vi "test1.vi"() -> ()   [LabVIEW 2014]
uses:
  <userlib>/ROS for LabVIEW Software/ROS/Code/Console/Servers/ServerSubs/TopicDef.ctl
  <userlib>/ROS for LabVIEW Software/ROS/Code/SubVIs/_ROSDirection.ctl
  <userlib>/ROS for LabVIEW Software/ROS/MessageBuilding/std_msgs/subs/float32Scalar.vi
  <userlib>/ROS for LabVIEW Software/ROS/MessageBuilding/std_msgs/subs/stringScalar.vi
  <userlib>/ROS for LabVIEW Software/ROS/MessageBuilding/std_msgs/subs/u8Scalar.vi
panel:
  in  "Stamp":cluster{"frame_id":string, "reset seq?":bool}={"frame_id"="base_range", "reset seq?"=FALSE}
  in  "Range Data":T1={"Radiation Type"=enum."ultrasound", "Field of View"=2.0, "Min Range (m)"=0.0, "Max Range (m)"=2.0, "Range (m)"=0.0}
  in  "Numeric":sgl
  in  "I said: 2":string="Hello world!"
  out "error out 2":errorcluster
  in  "stop 2":bool
  in  "I said:":string="Hello world!"
  out "error out":errorcluster
  in  "stop":bool
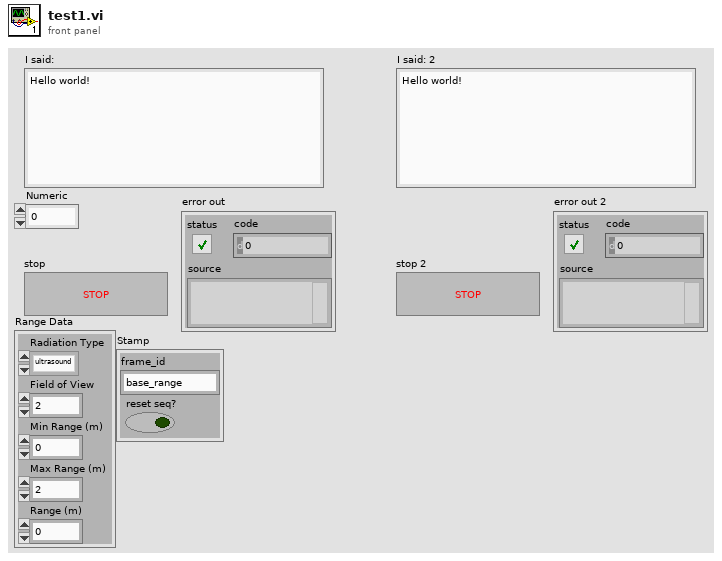
[diagram p1: front panel]
types:
  T1 = cluster{"Radiation Type":enum16{"ultrasound", "infrared"}, "Field of View":sgl, "Min Range (m)":sgl, "Max Range (m)":sgl, "Range (m)":sgl}
  T2 = typedef "TopicDef.ctl" = cluster{"Topic":string, "Type":string, "Action":T3, "Update (ms)":u16, "queue size":u16}
  T3 = typedef "_ROSDirection.ctl" = enum16{"Node", "Publisher", "Subscriber", "ServiceClient", "ServiceProvider"}
  T4 = typedef "_ROSControl.ctl" = cluster{"topic port":u16, "Node":string, "topic":string, "type":string, "node port":u16, "error ":errorcluster, "Direction":T3, "Update (ms)":u16, "FIFO size":u16}
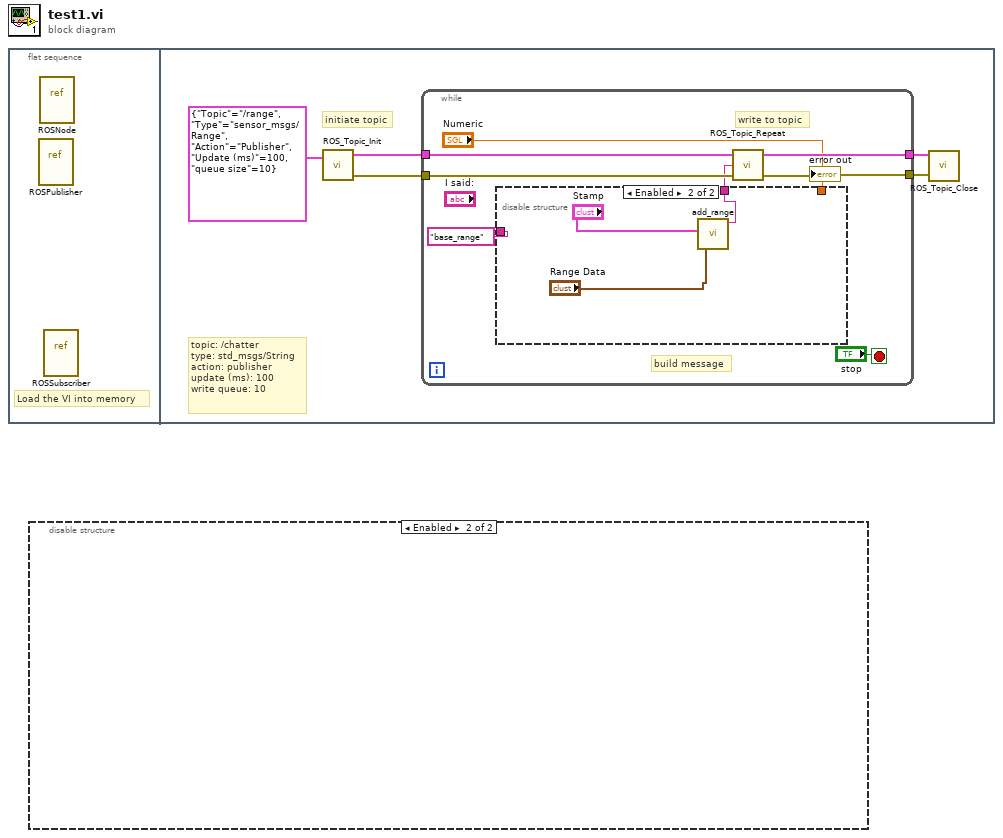
[diagram p0: block diagram]
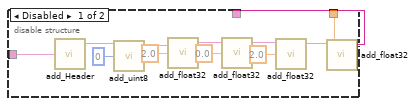
[diagram p2: hidden frame]
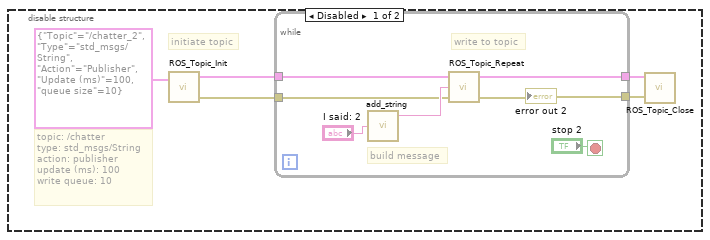
[diagram p3: hidden frame]
diagram:
  n1 = flat-sequence {
    frame #0 {
      # "Load the VI into memory"
      n2 = vi-ref <userlib>:"ROSPublisher.vi"() -> ()  [unwired: 1 out]
      n3 = vi-ref <userlib>:"ROSNode.vi"() -> ()  [unwired: 1 out]
      n4 = vi-ref <userlib>:"ROSSubscriber.vi"() -> ()  [unwired: 1 out]
    }
    frame #1 {
      # "initiate topic"
      # "topic: /chatter\ntype: std_msgs/String\naction: publisher\nupdate (ms): 100\nwrite queue: 10"
      n5 = call <userlib>:"ROS_Topic_Init.vi"("Definitions"=T2 {"Topic"="/range", "Type"="sensor_msgs/Range", "Action"=enum."Publisher", "Update (ms)"=100, "queue size"=10}) -> ("ROS out"=w4:T4, "error out"=w3:errorcluster)  [unwired: 2 in]
      n6 = while {
        tunnel: w4 -> [w13]
        tunnel: w3 -> [w12]
        tunnel: [w10] -> w2
        tunnel: [w9] -> w1
        stop <- "stop" stop-if-true
        # "build message"
        # "write to topic"
        n7 = disable-structure shown="Enabled" {
          disable-tunnel: "base_range" ("frame_id") -> [w25 _]
          disable-tunnel: "Numeric" -> [w15 _]
          disable-tunnel: [w14 w27] -> w6
          frame Disabled {
            n8 = call <userlib>:"add_Header.vi"("frame_id"=w25) -> ("msg out"=w24:string)  [unwired: 4 in]
            n9 = call-poly <userlib>:"add_uint8.vi"("Numeric"=u8 0, "msg in"=w24) -> ("msg out"=w22:string)  [unwired: 3 in]
            n10 = call-poly <userlib>:"add_float32.vi"("Numeric"=sgl 2.0, "msg in"=w22) -> ("msg out"=w20:string)  [unwired: 3 in]
            n11 = call-poly <userlib>:"add_float32.vi"("Numeric"=sgl 0.0, "msg in"=w20) -> ("msg out"=w19:string)  [unwired: 3 in]
            n12 = call-poly <userlib>:"add_float32.vi"("Numeric"=sgl 2.0, "msg in"=w19) -> ("msg out"=w16:string)  [unwired: 3 in]
            n13 = call-poly <userlib>:"add_float32.vi"("Numeric"=w15, "msg in"=w16) -> ("msg out"=w14:string)  [unwired: 3 in]
          }
          frame Enabled {
            n14 = call <userlib>:"add_range.vi"("Range Data"="Range Data", "Stamp"="Stamp") -> ("msg out"=w27:string)  [unwired: 5 in]
          }
        }
        n15 = call <userlib>:"ROS_Topic_Repeat.vi"("error in (no error)"=w12, "Msg in"=w6, "ROS in"=w13) -> ("error out"=w9:errorcluster, "ROS out"=w10:T4)  [unwired: 1 in]
        "error out" <- w9
      }
      n16 = call <userlib>:"ROS_Topic_Close.vi"("error in"=w1, "ROS in"=w2) -> ()  [unwired: 2 in, 1 out]
    }
  }
  n17 = disable-structure shown="Enabled" {
    frame Disabled {
      # "initiate topic"
      # "topic: /chatter\ntype: std_msgs/String\naction: publisher\nupdate (ms): 100\nwrite queue: 10"
      n18 = call <userlib>:"ROS_Topic_Init.vi"("Definitions"=T2 {"Topic"="/chatter_2", "Type"="std_msgs/String", "Action"=enum."Publisher", "Update (ms)"=100, "queue size"=10}) -> ("ROS out"=w32:T4, "error out"=w31:errorcluster)  [unwired: 2 in]
      n19 = while {
        tunnel: w32 -> [w40]
        tunnel: w31 -> [w37]
        tunnel: [w35] -> w30
        tunnel: [w34] -> w29
        stop <- "stop 2" stop-if-true
        # "build message"
        # "write to topic"
        n20 = call-poly <userlib>:"add_string.vi"("String"="I said: 2") -> ("msg out"=w38:string)  [unwired: 4 in]
        n21 = call <userlib>:"ROS_Topic_Repeat.vi"("error in (no error)"=w37, "Msg in"=w38, "ROS in"=w40) -> ("error out"=w34:errorcluster, "ROS out"=w35:T4)  [unwired: 1 in]
        "error out 2" <- w34
      }
      n22 = call <userlib>:"ROS_Topic_Close.vi"("error in"=w29, "ROS in"=w30) -> ()  [unwired: 2 in, 1 out]
    }
    frame Enabled {
    }
  }
